vi "testReposition.vi"() -> ()   [LabVIEW 2022 SP3]
panel:
  in  "y":dbl
  in  "x":dbl
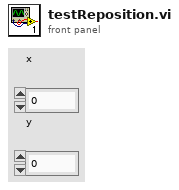
[diagram p1: front panel]
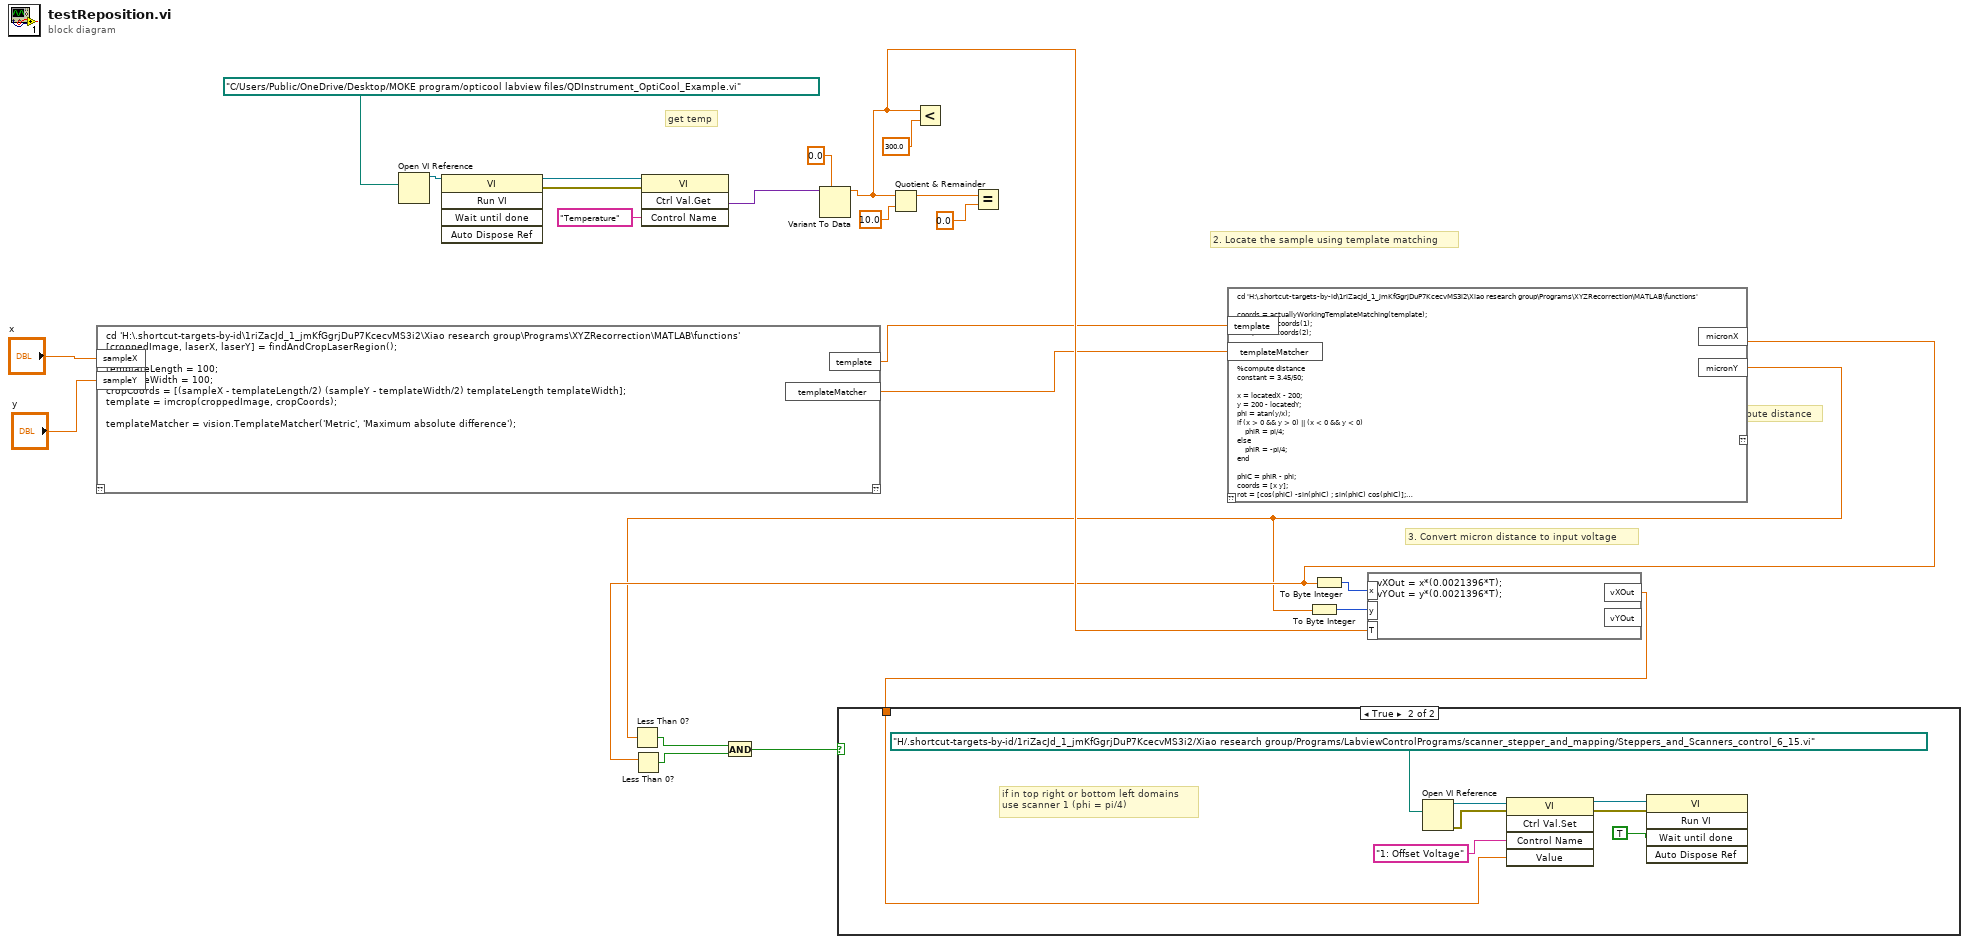
[diagram p0: block diagram]
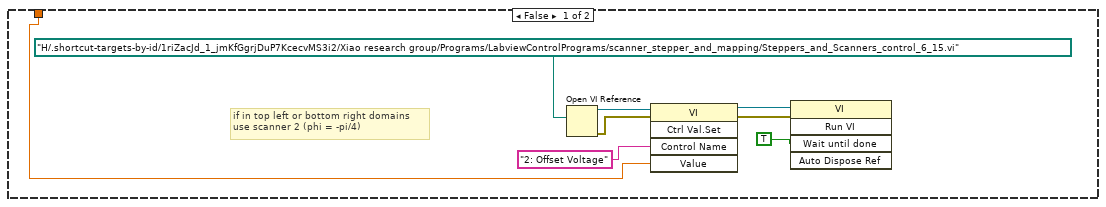
[diagram p2: hidden frame]
diagram:
  # "get temp"
  # "3. Convert micron distance to input voltage"
  # "compute distance"
  # "2. Locate the sample using template matching"
  n1 = script code="cd 'H:\\.shortcut-targets-by-id\\1riZacJd_1_jmKfGgrjDuP7KcecvMS3i2\\Xiao research group\\Programs\\XYZRecorrection\\MATLAB\\functions'\n[croppedImage, laserX, laserY] = findAndCropLaserRegion();\n\ntemplateLength = 100;\ntemplateWidth = 100;\ncropCoords = [(sampleX - templateLength/2) (sampleY - templateWidth/2) templateLength templateWidth];\ntemplate = imcrop(croppedImage, cropCoords);\n\ntemplateMatcher = vision.TemplateMatcher('Metric', 'Maximum absolute difference');"("sampleX"="x", "sampleY"="y") -> ("template"=w8:dbl, "templateMatcher"=w7:dbl)  [unwired: 1 in, 1 out]
  n2 = Open VI Reference(vi path=path "C:/Users/Public/OneDrive/Desktop/MOKE program/opticool labview files/QDInstrument_OptiCool_Example.vi") -> (vi reference=w17:refnum<vi>)  [unwired: 5 in, 1 out]
  n3 = invoke class="VI" method="Run VI"(reference=w17) -> (reference out=w18:refnum<vi>, error out=w19:errorcluster)  [unwired: 4 in, 3 out]
  n4 = invoke class="VI" method="Ctrl Val.Get"(reference=w18, error in=w19, "Control Name"="Temperature") -> ("Get Control Value Variant"=w20:variant)  [unwired: 1 in, 3 out]
  n5 = Variant To Data(type=0.0, Variant=w20) -> (data=w9:dbl)  [unwired: 1 in, 1 out]
  n6 = Quotient & Remainder(x=w9, y=10.0) -> (x-y*floor(x/y)=w11:dbl)  [unwired: 1 out]
  n7 = Less?(x=w9, y=300.0) -> ()  [unwired: 1 out]
  n8 = Equal?(x=w11, y=0.0) -> ()  [unwired: 1 out]
  n9 = script code="cd 'H:\\.shortcut-targets-by-id\\1riZacJd_1_jmKfGgrjDuP7KcecvMS3i2\\Xiao research group\\Programs\\XYZRecorrection\\MATLAB\\functions'\n\ncoords = actuallyWorkingTemplateMatching(template);\nsampleX = coords(1);\nsampleY = coords(2);\n\n\n\n%compute distance\nconstant = 3.45/50;\n\nx = locatedX - 200;\ny = 200 - locatedY;\nphi = atan(y/x);\nif (x > 0 && y > 0) || (x < 0 && y < 0)\n    phiR = pi/4;\nelse\n    phiR = -pi/4;\nend\n\nphiC = phiR - phi;\ncoords = [x y];\nrot = [cos(phiC) -sin(phiC) ; sin(phiC) cos(phiC)];\nresult = coords.*rot;\nres = sum(result, 2);\nxprime = res(1);\nyprime = res(2);\n\nxDiff = xprime - x;\nyDiff = yprime - y;\n\nnegativePhiCorrectionPixels = sqrt(xDiff^2 + yDiff^2);\npositivePhiCorrectionPixels = sqrt(xprime^2 + yprime^2);\n\nmicronX = constant*negativePhiCorrectionPixels; \nmicronY = constant*positivePhiCorrectionPixels;"("template"=w8, "templateMatcher"=w7) -> ("micronX"=w4:dbl, "micronY"=w2:dbl)  [unwired: 1 in, 1 out]
  n10 = Less Than 0?(x=w2) -> (x < 0?=w23:bool)
  n11 = Less Than 0?(x=w4) -> (x < 0?=w22:bool)
  n12 = And(x=w23, y=w22) -> (x .and. y?=w21:bool)
  n13 = To Byte Integer(number=w2) -> (8bit integer=w1:i8)
  n14 = To Byte Integer(number=w4) -> (8bit integer=w3:i8)
  n15 = formula code="vXOut = x*(0.0021396*T);\nvYOut = y*(0.0021396*T);"("x"=w3, "y"=w1, "T"=w9) -> ("vXOut"=w24:dbl)  [unwired: 1 out]
  n16 = case shown="True" w21 {
    tunnel: w24 -> [w25 w33]
    frame False {
      # "if in top left or bottom right domains\nuse scanner 2 (phi = -pi/4)"
      n17 = Open VI Reference(vi path=path "H:/.shortcut-targets-by-id/1riZacJd_1_jmKfGgrjDuP7KcecvMS3i2/Xiao research group/Programs/LabviewControlPrograms/scanner_stepper_and_mapping/Steppers_and_Scanners_control_6_15.vi") -> (vi reference=w29:refnum<vi>, error out=w30:errorcluster)  [unwired: 5 in]
      n18 = invoke class="VI" method="Ctrl Val.Set"(reference=w29, error in=w30, "Control Name"="2: Offset Voltage", "Value"=w25) -> (reference out=w27:refnum<vi>, error out=w26:errorcluster)  [unwired: 1 in, 3 out]
      n19 = invoke class="VI" method="Run VI"(reference=w27, error in=w26, "Wait until done"=TRUE ("Wait Until Done")) -> ()  [unwired: 2 in, 5 out]
    }
    frame True {
      # "if in top right or bottom left domains\nuse scanner 1 (phi = pi/4)"
      n20 = Open VI Reference(vi path=path "H:/.shortcut-targets-by-id/1riZacJd_1_jmKfGgrjDuP7KcecvMS3i2/Xiao research group/Programs/LabviewControlPrograms/scanner_stepper_and_mapping/Steppers_and_Scanners_control_6_15.vi") -> (vi reference=w37:refnum<vi>, error out=w38:errorcluster)  [unwired: 5 in]
      n21 = invoke class="VI" method="Ctrl Val.Set"(reference=w37, error in=w38, "Control Name"="1: Offset Voltage", "Value"=w33) -> (reference out=w35:refnum<vi>, error out=w34:errorcluster)  [unwired: 1 in, 3 out]
      n22 = invoke class="VI" method="Run VI"(reference=w35, error in=w34, "Wait until done"=TRUE ("Wait Until Done")) -> ()  [unwired: 2 in, 5 out]
    }
  }
